vi "updateGain.vi"(8 "error in (no error)":errorcluster, 10 "Pane":refnum<vi>, 11 "ICSettingsViewer in":refnum<class "ICSettingsViewer.lvclass">) -> (0 "error out":errorcluster, 2 "Pane out":refnum<vi>, 3 "ICSettingsViewer out":refnum<class "ICSettingsViewer.lvclass">)   [LabVIEW 2009, in "Views.lvlib" / "Camera.lvlib" / "ICSettingsViewer.lvclass"]
uses:
  ICSettingsViewer.lvclass
  ICSettingsViewer.lvclass/ICSettingsViewer.ctl
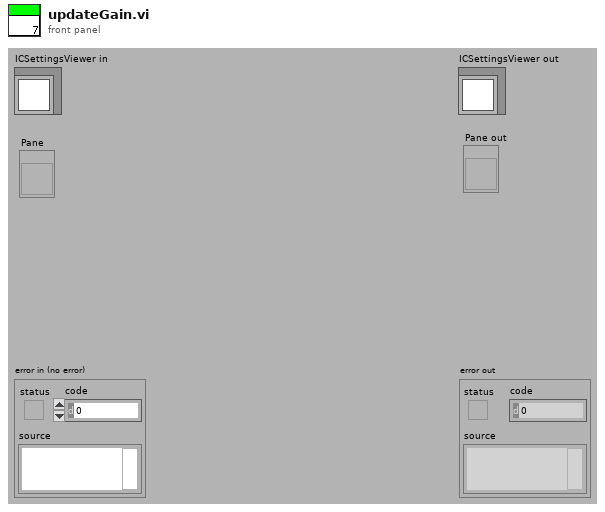
[diagram p1: front panel]
types:
  T1 = enum16{"exposure", "gain", "image_number", "Triggering", "start_trigger"}
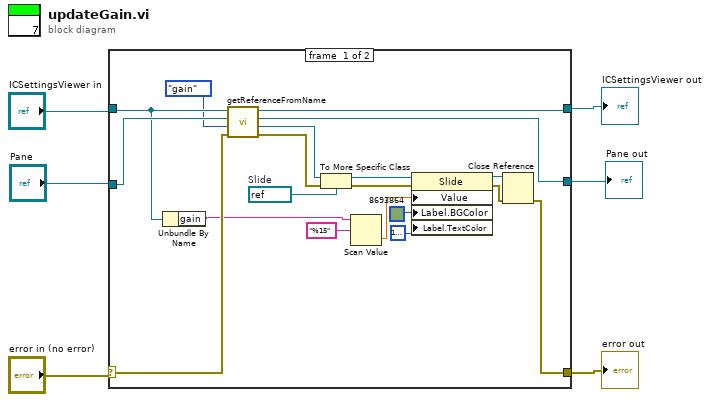
[diagram p0: block diagram]
diagram:
  n1 = case shown="No Error" "error in (no error)" {
    selector: "error in (no error)" -> [w23 w27]
    tunnel: [w11 w27] -> w5
    tunnel: [w24 w26] -> w3
    tunnel: "ICSettingsViewer in" -> [w16 w26]
    tunnel: "Pane" -> [w25 _]
    tunnel: [w22 _] -> w1
    frame #0 {
      w18 = refnum<vi> refnum  # Slide
      n2 = Unbundle By Name(w16) -> ("gain"=w10:string)
      n3 = call "getReferenceFromName.vi"("error in (no error)"=w23, "referenceName"=T1."gain", "Pane"=w25, "ICSettingsViewer in"=w16) -> ("error out"=w21:errorcluster, "Ctl Refnum"=w17:refnum<vi>, "Pane out"=w22:refnum<vi>, "ICSettingsViewer out"=w24:refnum<class "ICSettingsViewer.lvclass">)  [unwired: 3 in, 1 out]
      n4 = To More Specific Class(target class=w18, reference=w17, error in=w21) -> (specific class reference=w20:refnum<vi>, error out=w19:errorcluster)
      n5 = Scan Value(string=w10, format string="%15") -> (value=w14:dbl)  [unwired: 1 in, 1 out]
      n6 = property class="Slide"(reference=w20, error in=w19, "Value"=w14, "Label.BGColor"=u32 8693864, "Label.TextColor"=u32 16777222) -> (reference out=w13:refnum<vi>, error out=w12:errorcluster)
      n7 = Close Reference(reference=w13, error in (no error)=w12) -> (error out=w11:errorcluster)
    }
    frame #1 {
    }
  }
  "error out" <- w5
  "ICSettingsViewer out" <- w3
  "Pane out" <- w1
